vi "ReadHTMLFile.vi"(0 "file path (dialog if empty)":path, 2 "number of characters (all:-1)":i32=-1, 3 "start of read offset (chars.:0)":i32, 4 "advisory dialog? (display:T)":bool=TRUE, 5 "convert eol? (no:F)":bool) -> (6 "file path (NotAPath if cancelled)":path, 7 "contents":string, 9 "error out":errorcluster)   [LabVIEW 2016]
doc: "Reads a specified number of characters from a byte stream file beginning at a specified character offset."
panel:
  in  "prompt":string="Choose file to read."
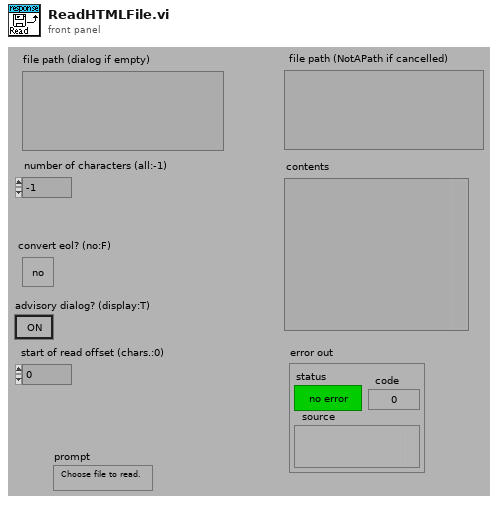
[diagram p1: front panel]
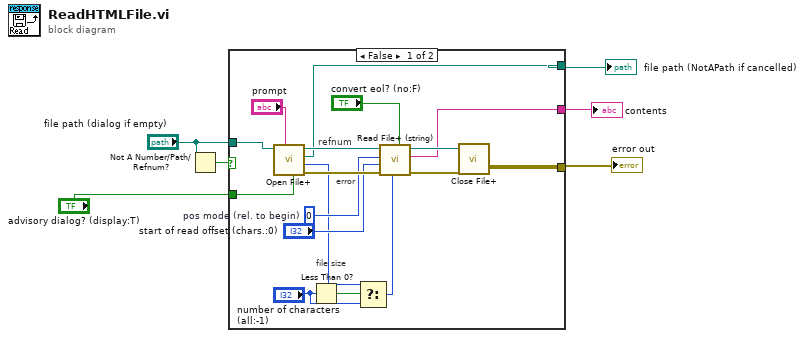
[diagram p0: block diagram]
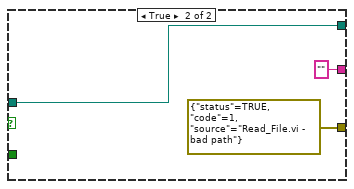
[diagram p2: hidden frame]
diagram:
  n1 = Not A Number/Path/Refnum?(number/path/refnum="file path (dialog if empty)") -> (NaN/Path/Refnum?=w2:bool)
  n2 = case shown="False" w2 {
    tunnel: [w17 w26] -> w6
    tunnel: [w10 errorcluster {"status"=TRUE, "code"=1, "source"="Read_File.vi - bad path"} ("error out")] -> w5
    tunnel: [w9 "" ("string")] -> w4
    tunnel: "file path (dialog if empty)" -> [w8 w26]
    tunnel: "advisory dialog? (display:T)" -> [w7 _]
    frame False {
      w22 = i16 0  # pos mode (rel. to begin)
      # "file size"
      # "error"
      # "refnum"
      n3 = call "Open File+.vi"("advisory dialog? (display:T)"=w7, "prompt"="prompt", "file path (\" \")"=w8) -> ("error out"=w23:errorcluster, "file size (bytes)"=w15:i32, "file path"=w17:path, "refnum"=w18:refnum<file>)  [unwired: 4 in, 1 out]
      n4 = Less Than 0?(x="number of characters (all:-1)") -> (x < 0?=w16:bool)
      n5 = Select(t=w15, s=w16, f="number of characters (all:-1)") -> (s? t:f=w13:i32)
      n6 = call "Read File+ (string).vi"("convert eol? (no:F)"="convert eol? (no:F)", "count"=w13, "error in (no error)"=w23, "pos offset (bytes:0)"="start of read offset (chars.:0)", "pos mode (rel. to current:2)"=w22, "refnum"=w18) -> ("error out"=w20:errorcluster, "string"=w9:string, "dup refnum"=w19:refnum<file>)  [unwired: 3 out]
      n7 = call "Close File+.vi"("error in (no error)"=w20, "refnum"=w19) -> ("error out"=w10:errorcluster)  [unwired: 5 out]
    }
    frame True {
    }
  }
  "file path (NotAPath if cancelled)" <- w6
  "contents" <- w4
  "error out" <- w5
